vi "OilWaterSeperate1.vi"(8 "error in (no error)":errorcluster, 9 "2D Picture":picture, 10 "Temp path":path, 11 "Image in":T2) -> (0 "error out":errorcluster, 1 "Oil Value":sgl, 2 "Water Value":sgl, 3 "Image Out":T2)   [LabVIEW 2012]
uses:
  <vilib>/vision/Image Controls.llb/IMAQ Image.ctl
  <vilib>/vision/NI_Vision_Development_Module.lvlib
panel:
  in  "Threshold Parameters":T1={"Level Type"=enum."Absolute Value", "Threshold Level"=128, "Hysteresis"=0}
  in  "Settings":T3={"Contrast"=40, "Filter width"=4, "Steepness"=2, "Subsampling Ratio"=5, "Show Search Area"=TRUE, "Show Search Lines"=TRUE, "Show Edges Found"=TRUE, "Show Result"=TRUE}
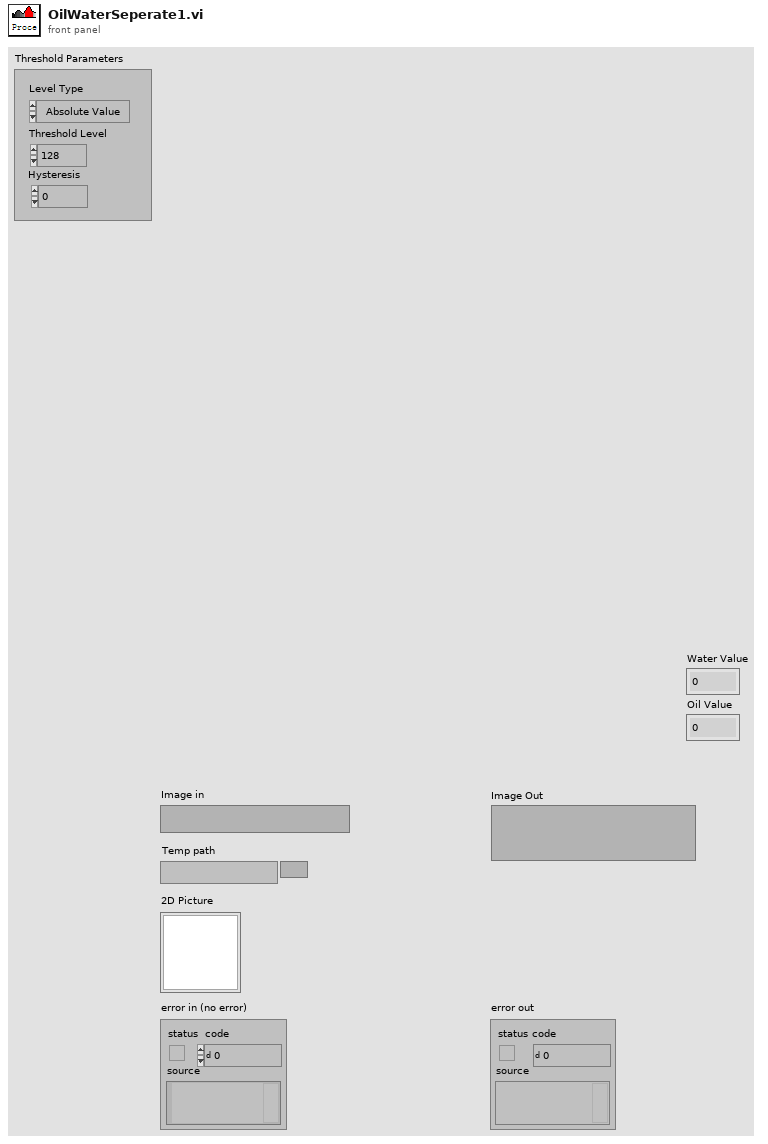
[diagram p1: front panel]
types:
  T1 = cluster{"Level Type":enum32{"Absolute Value", "Relative value"}, "Threshold Level":i32, "Hysteresis":i32}
  T2 = typedef "IMAQ Image.ctl" = refnum<image>
  T3 = cluster{"Contrast":i32, "Filter width":i32, "Steepness":i32, "Subsampling Ratio":u32, "Show Search Area":bool, "Show Search Lines":bool, "Show Edges Found":bool, "Show Result":bool}
  T4 = cluster{"Global Rectangle":i32[], "Contours":cluster{"ID":enum32{"External", "Internal"}, "Type":u32, "Coordinates":i32[]}[]}
  T5 = enum32{"Linear", "Log", "Exp", "Square", "Square root", "Power X", "Power 1/X"}
  T6 = cluster{"Position":cluster{"x":sgl, "y":sgl}, "Angle":sgl, "Scale":sgl, "Score":sgl, "Bounding Box":cluster{"x":sgl, "y":sgl}[]}[]
  T7 = cluster{"Position":cluster{"x":sgl, "y":sgl}, "Angle":sgl, "Scale":sgl, "Score":sgl, "Bounding Box":cluster{"x":sgl, "y":sgl}[]}
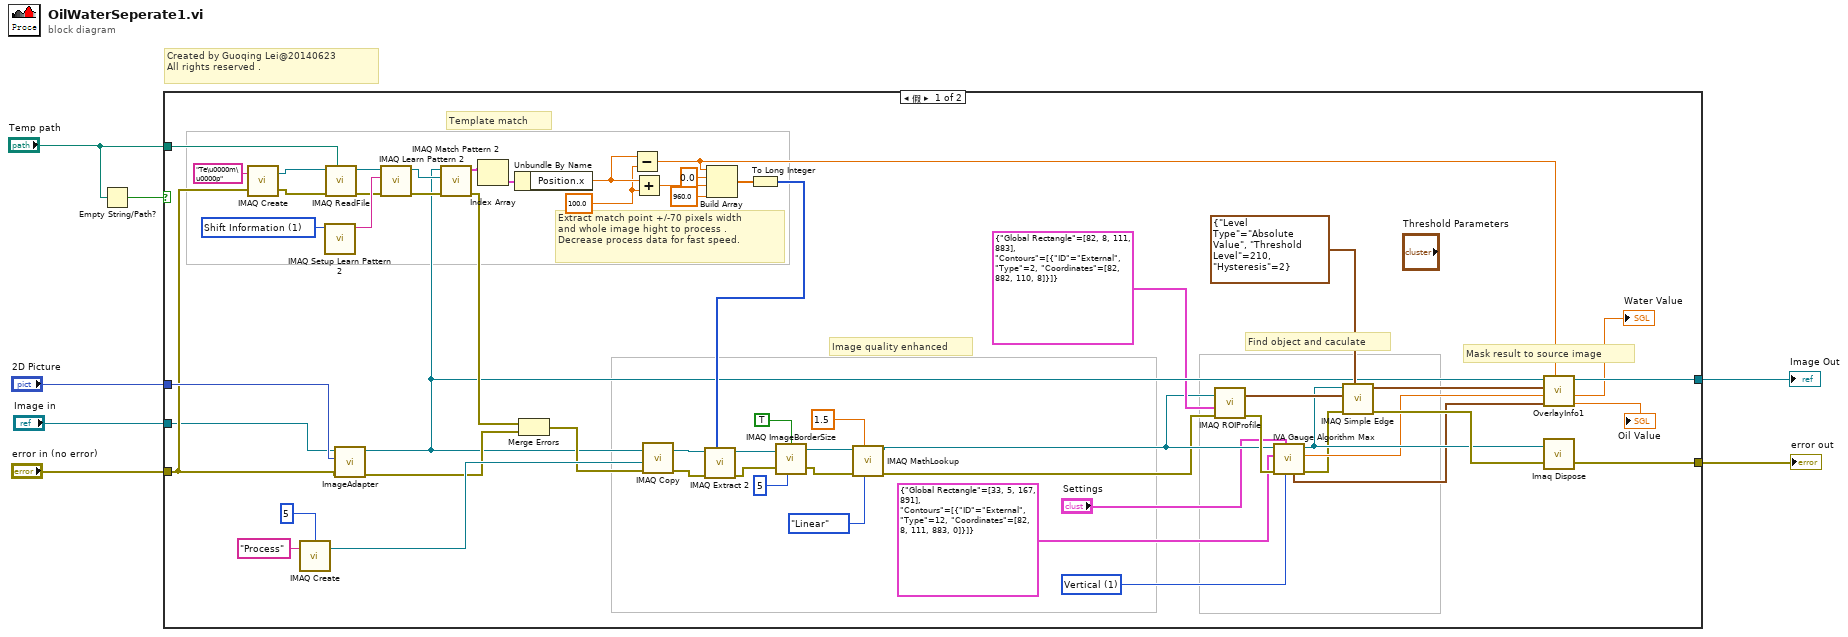
[diagram p0: block diagram]
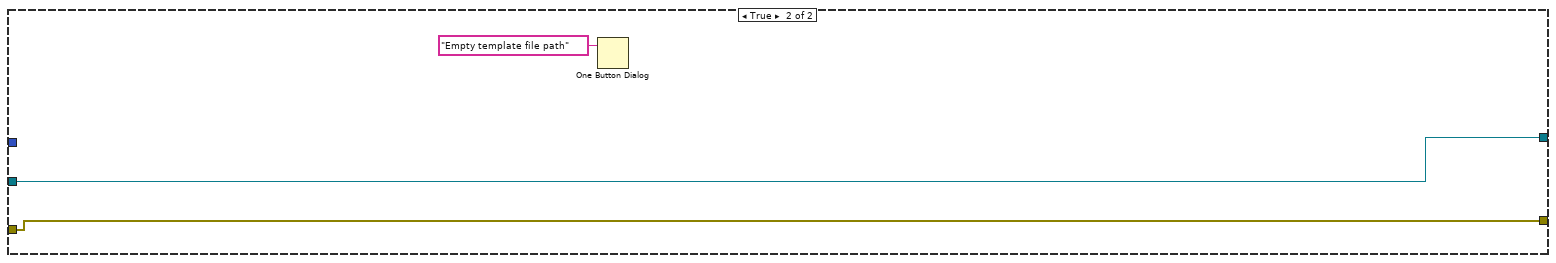
[diagram p2: hidden frame]
diagram:
  # "Created by Guoqing Lei@20140623 \nAll rights reserved ."
  n1 = Empty String/Path?(string/path="Temp path") -> (empty?=w6:bool)
  n2 = case shown="假" w6 {
    tunnel: "Temp path" -> [w48 _]
    tunnel: "2D Picture" -> [w29 _]
    tunnel: [w23 w68] -> w4
    tunnel: "error in (no error)" -> [w25 w68]
    tunnel: "Image in" -> [w24 w67]
    tunnel: [w22 w67] -> w1
    frame False {
      w43 = u16 1 items=["All", "Shift Information", "Rotation Information"] ("Learn Mode")
      w46 = u32 1 items=["Horizontal", "Vertical"] ("Scanning axis (Clamp (Rake) 1)")
      w53 = sgl 100.0 ("y")
      # "Extract match point +/-70 pixels width \nand whole image hight to process .\nDecrease process data for fast speed."
      # "Mask result to source image"
      # "Find object and caculate"
      # "Image quality enhanced"
      # "Template match"
      n3 = call "IMAQ Create"("Image Name"="Te\u0000m\u0000p", "error in (no error)"=w25) -> ("New Image"=w56:T2, "error out"=w57:errorcluster)  [unwired: 3 in]
      n4 = call "IMAQ Create"("Border Size"=5, "Image Name"="Process") -> ("New Image"=w36:T2)  [unwired: 3 in, 1 out]
      n5 = call "IMAQ Setup Learn Pattern 2"("Learn Mode"=w43) -> ("Learn Pattern Setup Data"=w44:string)  [unwired: 9 in, 1 out]
      n6 = call "IMAQ ReadFile"("File Path"=w48, "error in (no error)"=w57, "Image"=w56) -> ("error out"=w41:errorcluster, "Image Out"=w45:T2)  [unwired: 4 in, 3 out]
      n7 = call "ImageAdapter.vi"("error in (no error)"=w25, "2D Picture"=w29, "Image in"=w24) -> ("error out"=w27:errorcluster, "Image Out"=w16:T2)  [unwired: 7 in]
      n8 = call "IMAQ Learn Pattern 2"("error in (no error)"=w41, "Learn Pattern Setup Data"=w44, "Image"=w45) -> ("error out"=w40:errorcluster, "Template Image Out"=w39:T2)  [unwired: 7 in]
      n9 = call "IMAQ Match Pattern 2"("error in (no error)"=w40, "Template Image"=w39, "Image"=w16) -> ("error out"=w28:errorcluster, "Matches"=w42:T6)  [unwired: 6 in, 1 out]
      n10 = Index Array(array=w42) -> (element=w55:T7)  [unwired: 1 in]
      n11 = Unbundle By Name(w55) -> ("Position.x"=w54:sgl)
      n12 = Merge Errors(w28, w27) -> (w26:errorcluster)
      n13 = Subtract(x=w54, y=w53) -> (x-y=w38:sgl)
      n14 = Add(x=w54, y=w53) -> (x+y=w52:sgl)
      n15 = call "IMAQ Copy"("error in (no error)"=w26, "Image Dst"=w36, "Image Src"=w16) -> ("error out"=w30:errorcluster, "Image Dst Out"=w17:T2)  [unwired: 3 in]
      n16 = Build Array(w38, sgl 0.0 ("element"), w52, sgl 960.0 ("element")) -> (w32:sgl[])
      n17 = To Long Integer(number=w32) -> (32bit integer=w31:i32[])
      n18 = call "IMAQ Extract 2"("Optional Rectangle"=w31, "error in (no error)"=w30, "Image Src"=w17) -> ("error out"=w64:errorcluster, "Image Dst Out"=w51:T2)  [unwired: 7 in]
      n19 = call "IMAQ ImageBorderSize"("Get/Set Status? (Set)"=TRUE, "Image"=w51, "Image border size in"=5, "error in (no error)"=w64) -> ("Image Out"=w21:T2, "error out"=w20:errorcluster)  [unwired: 1 out]
      n20 = call "IMAQ MathLookup"("Operator"=T5."Linear", "X Value"=sgl 1.5, "error in (no error)"=w20, "Image Src"=w21) -> ("error out"=w12:errorcluster, "Image Dst Out"=w14:T2)  [unwired: 6 in]
      n21 = call "IMAQ ROIProfile"("error in (no error)"=w12, "ROI Descriptor"=T4 {"Global Rectangle"=[82, 8, 111, 883], "Contours"=[{"ID"=enum."External", "Type"=2, "Coordinates"=[82, 882, 110, 8]}]} ("ROI Descriptor (Edge Detector 1)"), "Image"=w14) -> ("error out"=w34:errorcluster, "Pixel Coordinates"=w61:cluster{"X":u32, "Y":u32}[])  [unwired: 4 out]
      n22 = call <vilib>:"IVA Gauge Algorithm Max.vi"("Scanning axis"=w46, "Settings"="Settings", "error in (no error)"=w34, "ROI Descriptor"=T4 {"Global Rectangle"=[33, 5, 167, 891], "Contours"=[{"ID"=enum."External", "Type"=12, "Coordinates"=[82, 8, 111, 883, 0]}]} ("ROI Descriptor (Max Clamp 1)"), "Image"=w14) -> ("error out"=w33:errorcluster, "Distance"=w37:sgl, "Image Out"=w47:T2, "Distance Points"=w13:cluster{"X":sgl, "Y":sgl}[])  [unwired: 1 in, 2 out]
      n23 = call "IMAQ Simple Edge"("Threshold Parameters"=T1 {"Level Type"=enum."Absolute Value", "Threshold Level"=210, "Hysteresis"=2} ("Threshold Parameters (Edge Detector 1)"), "error in (no error)"=w33, "Pixel Coordinates"=w61, "Image Src"=w47) -> ("error out"=w60:errorcluster, "Edges Coordinates"=w59:cluster{"X":sgl, "Y":sgl}[])  [unwired: 2 in, 4 out]
      n24 = call "OverlayInfo1.vi"("Offset"=w38, "Distance Points"=w13, "TotalDistance"=w37, "Edges Coordinates in"=w59, "Image in"=w16) -> ("Oil Value"=→"Oil Value":sgl, "Water Value"=→"Water Value":sgl, "Image Out"=w22:T2)  [unwired: 4 in]
      n25 = call "Imaq Dispose"("Image"=w47, "error in (no error)"=w60) -> ("error out"=w23:errorcluster)  [unwired: 4 in]
    }
    frame True {
      n26 = One Button Dialog(message="Empty template file path") -> ()  [unwired: 1 in, 1 out]
    }
  }
  "error out" <- w4
  "Image Out" <- w1
